vi "Add Glyph to Picture - Picture.vi"(4 "Mask Color (Black)":u32(colorbox), 5 "Position (0,0)":cluster{"Horizontal":i16, "Vertical":i16}, 6 "Glyph {picture}":picture, 7 "picture in":picture) -> (3 "picture out":picture)   [LabVIEW 2025, in "XNode Support.lvlib"]
doc: "Adds a glyph to an image at the specified point, interpreting the \"Mask Color\" as transparent.\nThe inputs of both the image in, and the glyph can be either a Picture, an Image Cluster, or a Pixmap."
uses:
  XNode Support.lvlib
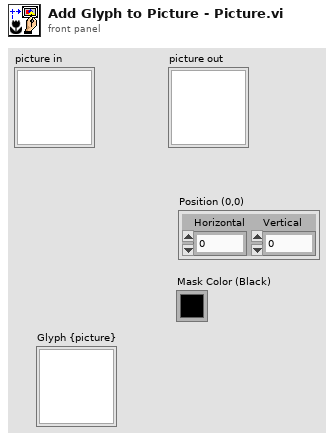
[diagram p1: front panel]
types:
  T1 = typedef "imagedata.ctl" = cluster{"image type":i32, "image depth":i32, "image":u8[], "mask":u8[], "colors":u32[], "Rectangle":cluster{"left":i16, "top":i16, "right":i16, "bottom":i16}}
  T2 = cluster{"Horizontal":i16, "Vertical":i16, "Horizontal":i16, "Vertical":i16}
  T3 = cluster{"left":i16, "top":i16, "right":i16, "bottom":i16}
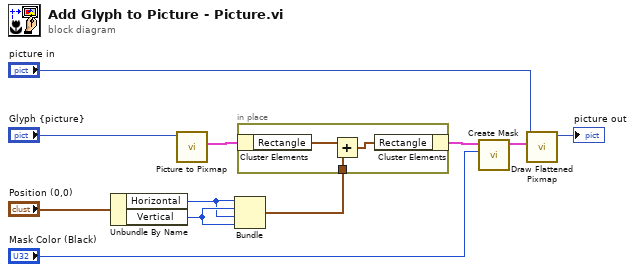
[diagram p0: block diagram]
diagram:
  n1 = Unbundle By Name("Position (0,0)") -> ("Horizontal"=w1:i16, "Vertical"=w7:i16)
  n2 = call <vilib>:"Picture to Pixmap.vi"("picture"="Glyph {picture}") -> ("image data"=w3:T1)  [unwired: 9 in, 1 out]
  n3 = Bundle("Horizontal"=w1, "Vertical"=w7, "Horizontal"=w1, "Vertical"=w7) -> (w5:T2)  [unwired: 1 in]
  n4 = in-place {
    in-place-border: w5 -> [w12]
    n5 = in-place-cluster #1(w3) -> ("Rectangle"=w14:T3)
    n6 = Add(x=w14, y=w12) -> (x+y=w13:cluster{i16, i16, i16, i16})
    n7 = in-place-cluster #1("Rectangle"=w13) -> (w11:T1)
  }
  n8 = call <vilib>:"Create Mask.vi"("Mask Color (Black)"="Mask Color (Black)", "image data"=w11) -> ("image data"=w9:T1)  [unwired: 9 in]
  n9 = call <vilib>:"Draw Flattened Pixmap.vi"("image data"=w9, "picture"="picture in") -> ("new picture"=→"picture out":picture)  [unwired: 7 in]
